vi "Smoother.vi"(8 "tolerance":dbl, 9 "B":dbl, 10 "A":dbl, 11 "Array In":dbl[][](array[numeric])) -> (3 "Array Out":dbl[][](array[numeric]))   [LabVIEW 2016]
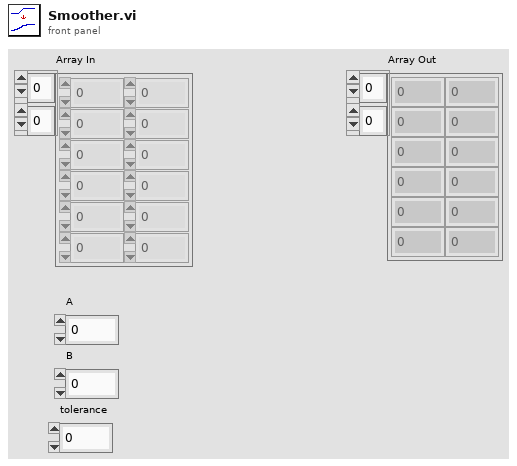
[diagram p1: front panel]
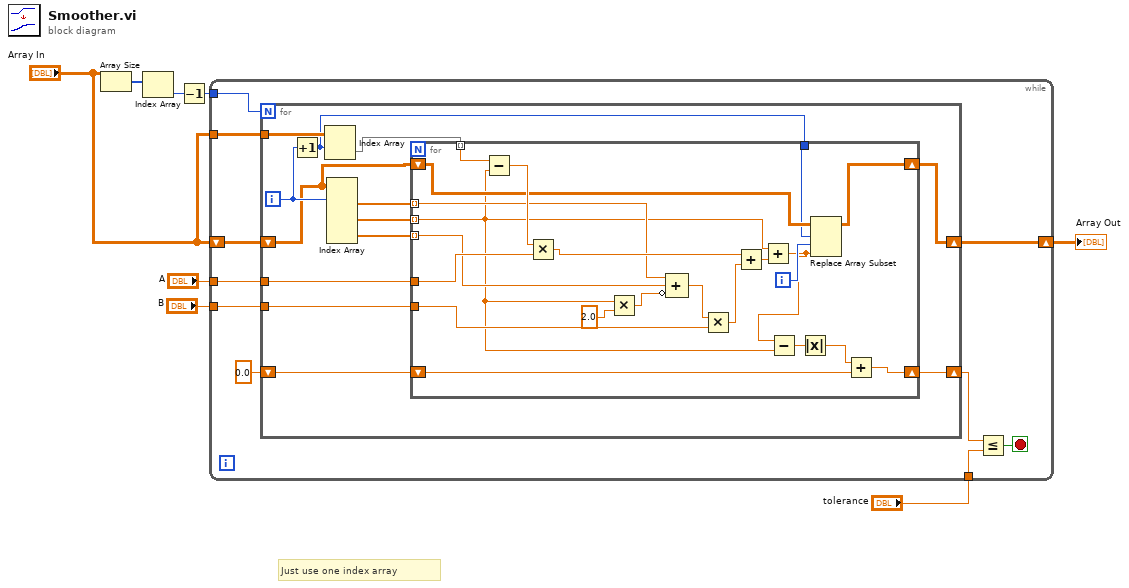
[diagram p0: block diagram]
diagram:
  # "Just use one index array"
  n1 = Array Size(array="Array In") -> (size(s)=w8:i32[])
  n2 = Index Array(array=w8) -> (element=w7:i32)  [unwired: 1 in]
  n3 = Decrement(x=w7) -> (x-1=w6:i32)
  n4 = while {
    tunnel: w6 -> [w18]
    tunnel: "A" -> [w17]
    tunnel: "B" -> [w16]
    tunnel: "Array In" -> [w15]
    shift-right: [w13] -> w1
    shift-left: "Array In" -> [w14]
    tunnel: "tolerance" -> [w12]
    stop <- w11 stop-if-true
    n5 = for {
      N: w18 -> [_]
      tunnel: w17 -> [w31]
      tunnel: w16 -> [w30]
      tunnel: w15 -> [w28]
      shift-right: [w21] -> w13
      shift-left: w14 -> [w23]
      shift-right: [w20] -> w9
      shift-left: 0.0 -> [w19]
      i -> [w27]
      n6 = Increment(x=w27) -> (x+1=w22:i32)
      n7 = Index Array(array=w28, index (row)=w22) -> (element=w26:dbl[])  [unwired: 1 in]
      n8 = Index Array(array=w23, index (row) #1=w27) -> (element #1=w25:dbl[], element #2=w29:dbl[], element #3=w24:dbl[])  [unwired: 5 in]
      n9 = for {
        tunnel: w29 -> [w36] mode=indexing
        tunnel: w31 -> [w53]
        tunnel: w30 -> [w49]
        tunnel: w26 -> [w52] mode=indexing
        tunnel: w25 -> [w48] mode=indexing
        tunnel: w24 -> [w47] mode=indexing
        tunnel: w22 -> [w39]
        shift-right: [w38] -> w21
        shift-left: w23 -> [w41]
        shift-right: [w34] -> w20
        shift-left: w19 -> [w33]
        i -> [w40]
        n10 = Subtract(x=w52, y=w36) -> (x-y=w51:dbl)
        n11 = Multiply(x=w51, y=w53) -> (x*y=w50:dbl)
        n12 = Multiply(x=w36, y=2.0) -> (x*y=w46:dbl)
        n13 = Compound Arithmetic op=ADD(w48, w47, invert w46) -> (w44:dbl)
        n14 = Multiply(x=w44, y=w49) -> (x*y=w43:dbl)
        n15 = Add(x=w50, y=w43) -> (x+y=w42:dbl)
        n16 = Add(x=w36, y=w42) -> (x+y=w37:dbl)
        n17 = Subtract(x=w37, y=w36) -> (x-y=w35:dbl)
        n18 = Absolute Value(x=w35) -> (abs(x)=w32:dbl)
        n19 = Replace Array Subset(array=w41, new element=w37, index (row)=w39, index (col)=w40) -> (w38:dbl[][])
        n20 = Add(x=w32, y=w33) -> (x+y=w34:dbl)
      }
    }
    n21 = Less Or Equal?(x=w9, y=w12) -> (x <= y?=w11:bool)
  }
  "Array Out" <- w1
